vi "写入通信设置.vi"(8 "error in (no error)":errorcluster, 10 "通信设置":cluster{"本地端口":u16, "最大字节数/读取":i32}={"本地端口"=1024, "最大字节数/读取"=548}, 11 "串口通信类 in":refnum<class "串口通信类.lvclass">) -> (0 "error out":errorcluster, 3 "串口通信类 out":refnum<class "串口通信类.lvclass">)   [LabVIEW 2015, in "串口通信类.lvclass"]
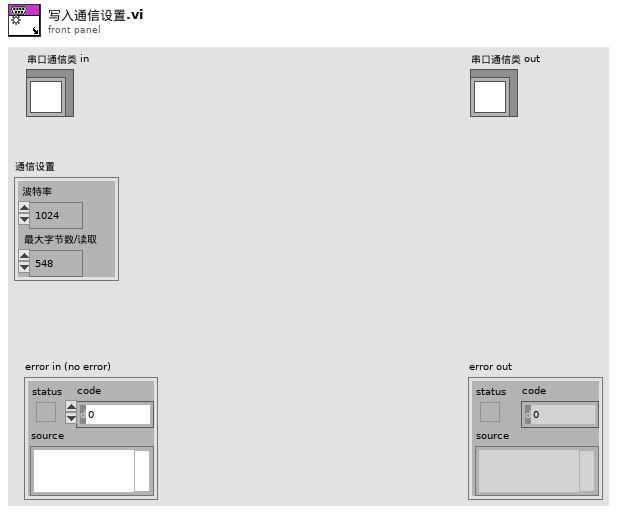
[diagram p1: front panel]
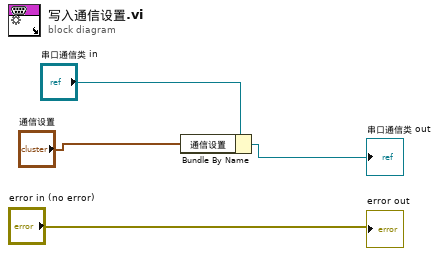
[diagram p0: block diagram]
diagram:
  n1 = Bundle By Name(cluster="串口通信类 in", "通信设置"="通信设置") -> (→"串口通信类 out":refnum<class "串口通信类.lvclass">)
  "error out" <- "error in (no error)"
